vi "extract_ollama_embeddings.vi"(10 "body":string, 11 "headers":string) -> (0 "error out":errorcluster, 3 "vector response":refnum<class "message_vectors.lvclass">)   [LabVIEW 2020, in "llm_ollama_embedding.lvclass"]
uses:
  llm_ollama_embedding.lvclass
  message_vectors/message_vectors.lvclass
  message_vectors/embedding.ctl
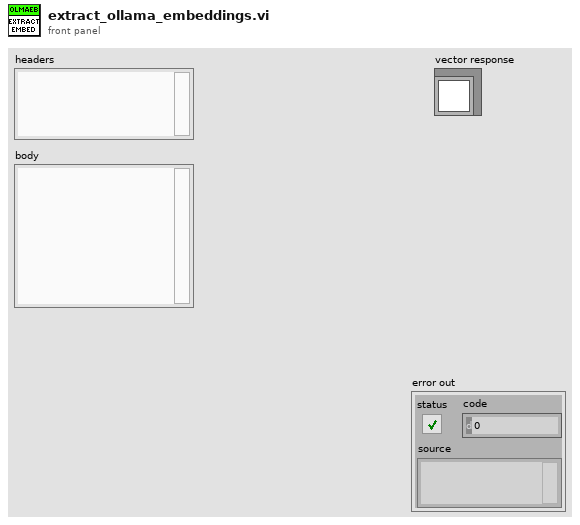
[diagram p1: front panel]
types:
  T1 = typedef "message_vectors.lvclass/embedding.ctl" = cluster{"index":u32, "Vectors":dbl[]}
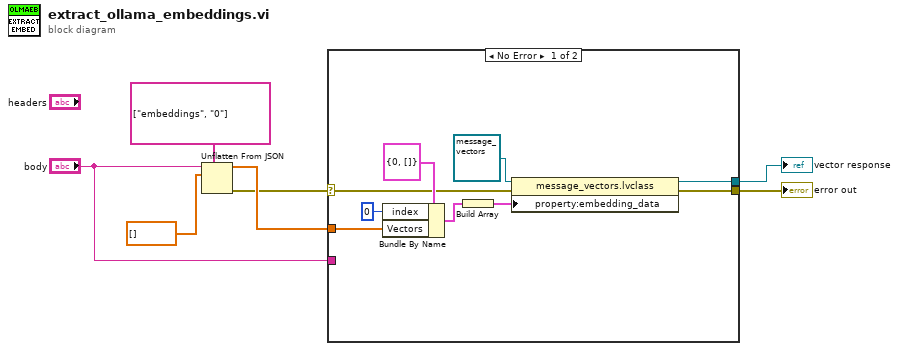
[diagram p0: block diagram]
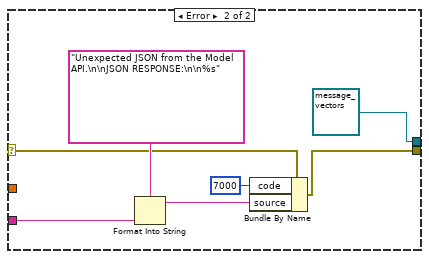
[diagram p2: hidden frame]
diagram:
  n1 = Unflatten From JSON(path=string[] ["embeddings", "0"], JSON string="body", type and defaults=dbl[] []) -> (value=w5:dbl[], error out=w4:errorcluster)  [unwired: 4 in]
  n2 = case shown="No Error" w4 {
    selector: w4 -> [w8 w17]
    tunnel: w5 -> [w14 _]
    tunnel: [w10 w19] -> w3
    tunnel: [w9 refnum<class "message_vectors.lvclass"> refnum ("message_vectors.lvclass")] -> w2
    tunnel: "body" -> [_ w20]
    frame No Error {
      n3 = Bundle By Name(cluster=T1 {"index"=0, "Vectors"=[]} ("embedding"), "index"=u32 0, "Vectors"=w14) -> (w12:T1)
      n4 = Build Array(w12) -> (w11:T1[])
      n5 = property class="message_vectors.lvclass"(reference=refnum<class "message_vectors.lvclass"> refnum ("message_vectors.lvclass"), error in=w8, "property:embedding_data"=w11) -> (reference out=w9:refnum<class "message_vectors.lvclass">, error out=w10:errorcluster)
    }
    frame Error {
      n6 = Format Into String(format string="Unexpected JSON from the Model API.\n\nJSON RESPONSE:\n\n%s", w20) -> (resulting string=w22:string)  [unwired: 2 in, 1 out]
      n7 = Bundle By Name(cluster=w17, "code"=7000, "source"=w22) -> (w19:errorcluster)
    }
  }
  "vector response" <- w2
  "error out" <- w3
